vi "Initialize.vi"(8 "error in (no error)":errorcluster, 11 "Configuration in":refnum<class "Configuration.lvclass">) -> (0 "error out":errorcluster, 3 "Configuration out":refnum<class "Configuration.lvclass">)   [LabVIEW 2023, in "Configuration.lvlib" / "Configuration.lvclass"]
doc: "<b>Initialize</b>\nThis routine is implemented in the Pre-Launch Init override -> as a result, it is not necessary to call initialize anywhere else, and any methods that need to be called after post-launch intiialize can be implemented here.\n\n<b>Engine</b> - Calls Check for Errors"
uses:
  Library/Configuration.lvclass
  Library/Configuration.lvclass/Configuration.ctl
  builds/Framework/Engine.lvlibp/Managed Actor/Library/Managed Actor.lvclass
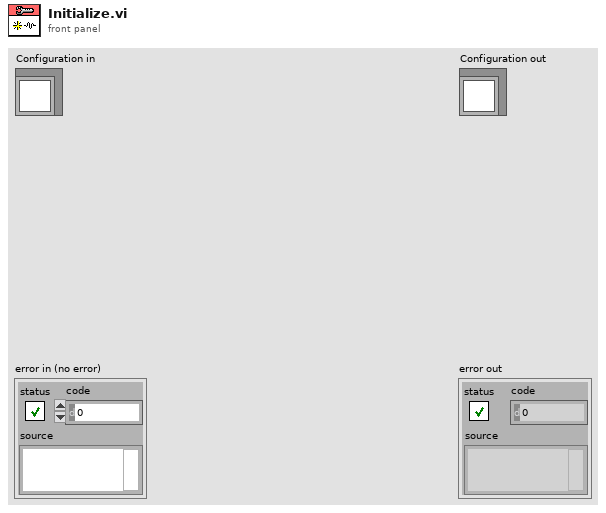
[diagram p1: front panel]
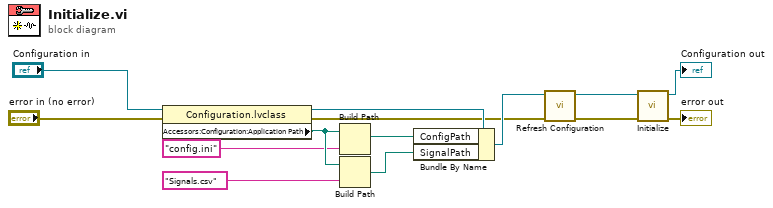
[diagram p0: block diagram]
diagram:
  n1 = property class="Configuration.lvclass"(reference="Configuration in", error in="error in (no error)") -> (reference out=w10:refnum<class "Configuration.lvclass">, error out=w2:errorcluster, "Accessors:Configuration:Application Path"=w9:path)
  n2 = Build Path(base path=w9, name or relative path="config.ini") -> (appended path=w6:path)
  n3 = Build Path(base path=w9, name or relative path="Signals.csv") -> (appended path=w5:path)
  n4 = Bundle By Name(cluster=w10, "ConfigPath"=w6, "SignalPath"=w5) -> (w4:refnum<class "Configuration.lvclass">)
  n5 = call "Refresh Configuration.vi"("error in (no error)"=w2, "Configuration in"=w4) -> ("error out"=w1:errorcluster, "Configuration out"=w3:refnum<class "Configuration.lvclass">)  [unwired: 8 in]
  n6 = call-parent "Initialize.vi"("error in (no error)"=w1, "Engine in"=w3) -> ("error out"=→"error out":errorcluster, "Engine out"=→"Configuration out":refnum<class "Configuration.lvclass">)  [unwired: 8 in]
